vi "Sensifier.vi"(10 "Array":string[](array[string])) -> (1 "Has Errors?":bool, 2 "Sensed":string[](array[string]))   [LabVIEW 2014]
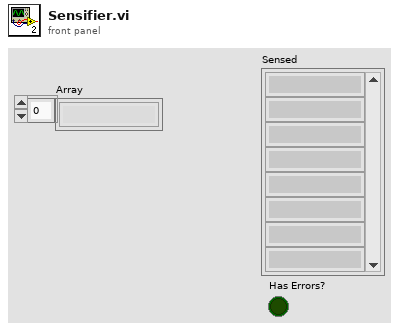
[diagram p1: front panel]
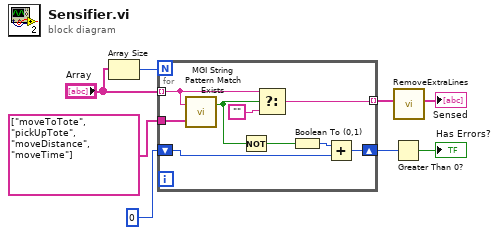
[diagram p0: block diagram]
diagram:
  n1 = Array Size(array="Array") -> (size(s)=w6:i32)
  n2 = for {
    N: w6 -> [_]
    tunnel: "Array" -> [w11] mode=indexing
    tunnel: string[] ["moveToTote", "pickUpTote", "moveDistance", "moveTime"] ("string array") -> [w17]
    tunnel: [w16] -> w2 mode=indexing
    shift-right: [w15] -> w5
    shift-left: i16 0 -> [w14]
    n3 = call <userlib>:"MGI String Pattern Match Exists.vi"("Patterns to Try"=w17, "String"=w11) -> ("Match Found"=w9:bool)  [unwired: 1 out]
    n4 = Not(x=w9) -> (.not. x?=w10:bool)
    n5 = Select(t=w11, s=w9, f="") -> (s? t:f=w16:string)
    n6 = Boolean To (0,1)(Boolean=w10) -> (0, 1=w13:i16)
    n7 = Add(x=w13, y=w14) -> (x+y=w15:i16)
  }
  n8 = Greater Than 0?(x=w5) -> (x > 0?=→"Has Errors?":bool)
  n9 = call "RemoveExtraLines.vi"("Sensed"=w2) -> ("Output"=→"Sensed":string[])  [unwired: 10 in]
